vi "LIN Polynom Ordnung je Komponente für Protokoll.vi"(6 "Aktion":T3, 8 "error in (no error)":errorcluster caption="Fehler (Eingang, kein Fehler)", 9 "Polynom-Ordnung view only":T1, 10 "Index in":T2, 11 "Polynom-Ordnung":T1) -> (0 "error out":errorcluster caption="Fehler (Ausgang)", 1 "Polynom-Ordnung view only out":T1, 2 "Index out":T2, 3 "Polynom-Ordnung out":T1, 4 "Polynom Ordnungen SPAN":T1[](array[typedef]), 5 "Polynom Ordnungen":T1[][](array[typedef]), 7 "Polynom Ordnungen view only":T1[][](array[typedef]))   [LabVIEW 2020, in "Linearisierung v2.lvlib" / "Protokoll.lvlib"]
uses:
  Protokoll.lvlib
  Auswahl Polynom Ordnung.ctl
  Linearisierung v2.lvlib
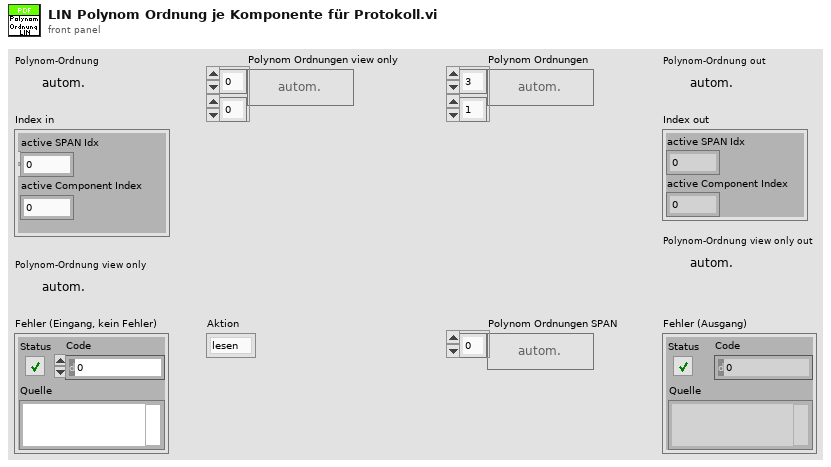
[diagram p1: front panel]
types:
  T1 = typedef "Linearisierung v2.lvlib/Auswahl Polynom Ordnung.ctl" = enum16{"autom.", "raw", "actual", "1", "2", "3", "4"}
  T2 = cluster{"active SPAN Idx":i32, "active Component Index":i32}
  T3 = typedef "Linearisierung v2.lvlib/Protokoll.lvlib/Aktion LIN Polynom Ordnung je Komponente für Protokoll.ctl" = enum16{"lesen", "schreiben", "init", "schreiben viewonly", "init initial"}
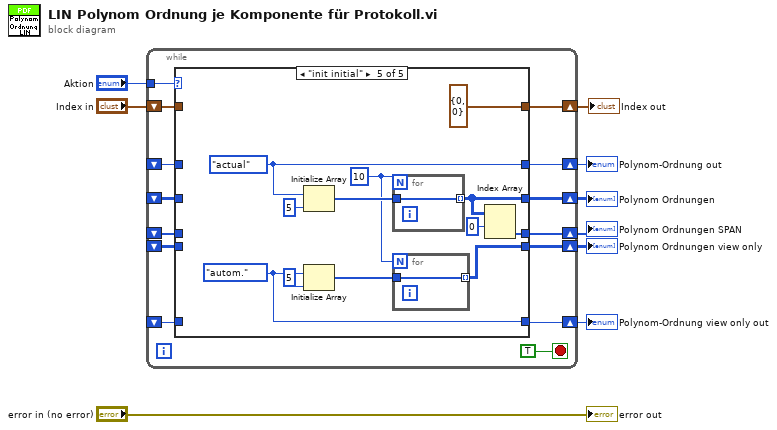
[diagram p0: block diagram]
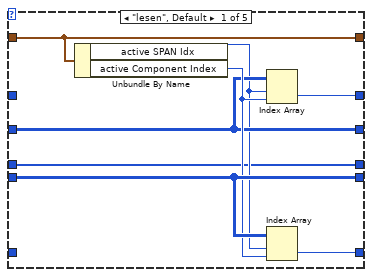
[diagram p2: hidden frame]
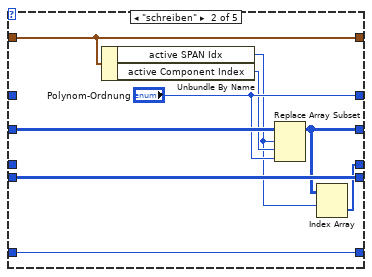
[diagram p3: hidden frame]
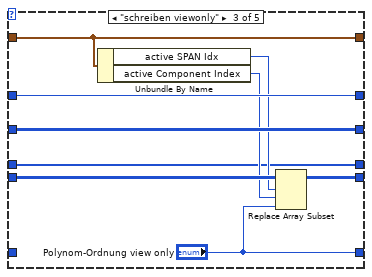
[diagram p4: hidden frame]
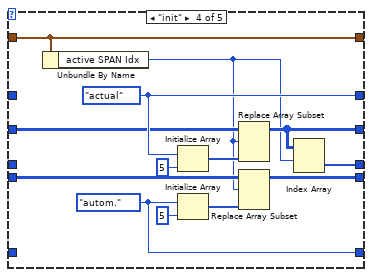
[diagram p5: hidden frame]
diagram:
  n1 = while {
    tunnel: "Aktion" -> [w22]
    shift-right: [w21] -> w8
    shift-left: "Index in" -> [w20]
    shift-right: [w19] -> w5
    shift-left: _ -> [w18]
    shift-right: [w17] -> w7
    shift-left: _ -> [w16]
    shift-right: [w15] -> w4
    shift-left: _ -> [w14]
    shift-right: [w13] -> w3
    shift-left: _ -> [w12]
    shift-right: [w11] -> w1
    shift-left: _ -> [w10]
    stop <- TRUE stop-if-true
    n2 = case shown="\"init initial\"" w22 {
      tunnel: [w27 w35 w42 w58 T2 {"active SPAN Idx"=0, "active Component Index"=0} ("Index in")] -> w21
      tunnel: w20 -> [w27 w35 w42 w58 _]
      tunnel: [w31 "Polynom-Ordnung" w48 w60 w72] -> w19
      tunnel: w18 -> [_ _ w48 _ _]
      tunnel: [w26 w34 w49 w52 w65] -> w17
      tunnel: w16 -> [w26 w40 w49 w57 _]
      tunnel: [w30 w38 w45 w55 w68] -> w15
      tunnel: w14 -> [w30 w38 w46 w54 _]
      tunnel: [w29 w37 "Polynom-Ordnung view only" w59 w71] -> w13
      tunnel: w12 -> [_ w37 _ _ _]
      tunnel: [w24 w32 w41 w50 w64] -> w11
      tunnel: w10 -> [w24 _ w41 _ _]
      frame "lesen", Default {
        n3 = Unbundle By Name(w27) -> ("active SPAN Idx"=w25:i32, "active Component Index"=w28:i32)
        n4 = Index Array(array=w26, index (row)=w25, index (col)=w28) -> (element=w31:T1)
        n5 = Index Array(array=w30, index (row)=w25, index (col)=w28) -> (element=w29:T1)
      }
      frame "schreiben" {
        n6 = Unbundle By Name(w35) -> ("active SPAN Idx"=w33:i32, "active Component Index"=w36:i32)
        n7 = Replace Array Subset(array=w40, new element="Polynom-Ordnung", index (row)=w33, index (col)=w36) -> (w34:T1[][])
        n8 = Index Array(array=w34, index (row)=w33) -> (element=w32:T1[])  [unwired: 1 in]
      }
      frame "schreiben viewonly" {
        n9 = Unbundle By Name(w42) -> ("active SPAN Idx"=w44:i32, "active Component Index"=w43:i32)
        n10 = Replace Array Subset(array=w46, new element="Polynom-Ordnung view only", index (row)=w44, index (col)=w43) -> (w45:T1[][])
      }
      frame "init" {
        w59 = Auswahl_Polynom_Ordnung."autom." ("Polynom-Ordnung")
        w60 = Auswahl_Polynom_Ordnung."actual" ("Polynom-Ordnung")
        n11 = Unbundle By Name(w58) -> ("active SPAN Idx"=w51:i32)
        n12 = Initialize Array(w60, 5 ("Dimensionsgröße")) -> (w56:T1[])
        n13 = Initialize Array(w59, 5 ("Dimensionsgröße")) -> (w53:T1[])
        n14 = Replace Array Subset(array=w57, new element=w56, index (row)=w51) -> (w52:T1[][])  [unwired: 1 in]
        n15 = Replace Array Subset(array=w54, new element=w53, index (row)=w51) -> (w55:T1[][])  [unwired: 1 in]
        n16 = Index Array(array=w52, index (row)=w51) -> (element=w50:T1[])  [unwired: 1 in]
      }
      frame "init initial" {
        w66 = 10
        w71 = Auswahl_Polynom_Ordnung."autom." ("Polynom-Ordnung")
        w72 = Auswahl_Polynom_Ordnung."actual" ("Polynom-Ordnung")
        n17 = Initialize Array(w72, 5 ("Dimensionsgröße")) -> (w70:T1[])
        n18 = Initialize Array(w71, 5 ("Dimensionsgröße")) -> (w69:T1[])
        n19 = for {
          N: w66 -> [_]
          tunnel: w70 -> [w76]
          tunnel: [w76] -> w65 mode=indexing
        }
        n20 = for {
          N: w66 -> [_]
          tunnel: w69 -> [w75]
          tunnel: [w75] -> w68 mode=indexing
        }
        n21 = Index Array(array=w65, index (row)=0 ("Index (Zeile)")) -> (element=w64:T1[])  [unwired: 1 in]
      }
    }
  }
  "Polynom Ordnungen" <- w7
  "Polynom-Ordnung out" <- w5
  "Polynom Ordnungen view only" <- w4
  "Polynom-Ordnung view only out" <- w3
  "Index out" <- w8
  "Polynom Ordnungen SPAN" <- w1
  "error out" <- "error in (no error)"
